vi "ke37xx Configure Channel Connection.vi"(0 "VISA Resource Name":refnum<visa-resource-name>, 5 "Connect Sequential (False)":bool, 7 "Connection Rule (0: None)":T1(ring), 11 "error in (no error)":errorcluster) -> (4 "VISA Resource Name Out":refnum<visa-resource-name>, 15 "error out":errorcluster)   [LabVIEW 2009, in "Keithley 3700 Series.lvlib"]
doc: "This VI allows you to configure the connection rule for channels as well as whether or not connections are closed sequentiall."
uses:
  <instrlib>/Keithley 3706/Keithley 3700 Series.lvlib
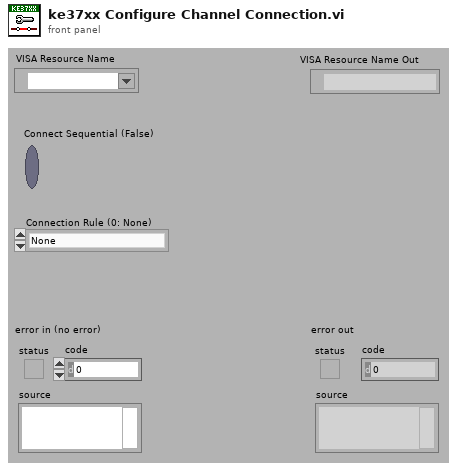
[diagram p1: front panel]
types:
  T1 = enum16{"None", "Make Before Break", "Break Before Make"}
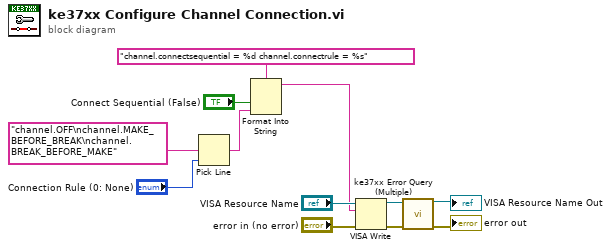
[diagram p0: block diagram]
diagram:
  n1 = Pick Line(multi-line string="channel.OFF\nchannel.MAKE_BEFORE_BREAK\nchannel.BREAK_BEFORE_MAKE", line index="Connection Rule (0: None)") -> (output string=w3:string)  [unwired: 1 out]
  n2 = Format Into String(format string="channel.connectsequential = %d channel.connectrule = %s", "Connect Sequential (False)", w3) -> (resulting string=w7:string)  [unwired: 2 in, 1 out]
  n3 = VISA Write(VISA resource name="VISA Resource Name", write buffer=w7, error in (no error)="error in (no error)") -> (VISA resource name out=w6:refnum<visa-resource-name>, error out=w5:errorcluster)  [unwired: 1 out]
  n4 = call <instrlib>:"ke37xx Error Query (Multiple).vi"("VISA resource name"=w6, "error in (no error)"=w5) -> ("VISA resource name out"=→"VISA Resource Name Out":refnum<visa-resource-name>, "error out"=→"error out":errorcluster)  [unwired: 12 out]
